vi "save data.vi"(8 "backwashing?":bool, 9 "coagulant dose":dbl) -> ()   [LabVIEW 2019]
uses:
  data buffer cmd.ctl
  file paths.ctl
panel:
  out "data labels":string[](array[string])
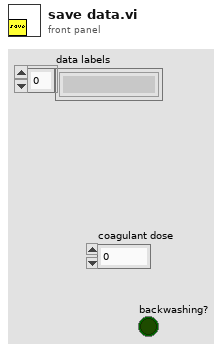
[diagram p1: front panel]
types:
  T1 = typedef "file paths.ctl" = enum16{"read paths", "close"}
  T2 = typedef "data buffer cmd.ctl" = enum16{"set buffer size", "write", "refill buffer", "read recent", "read all", "clear"}
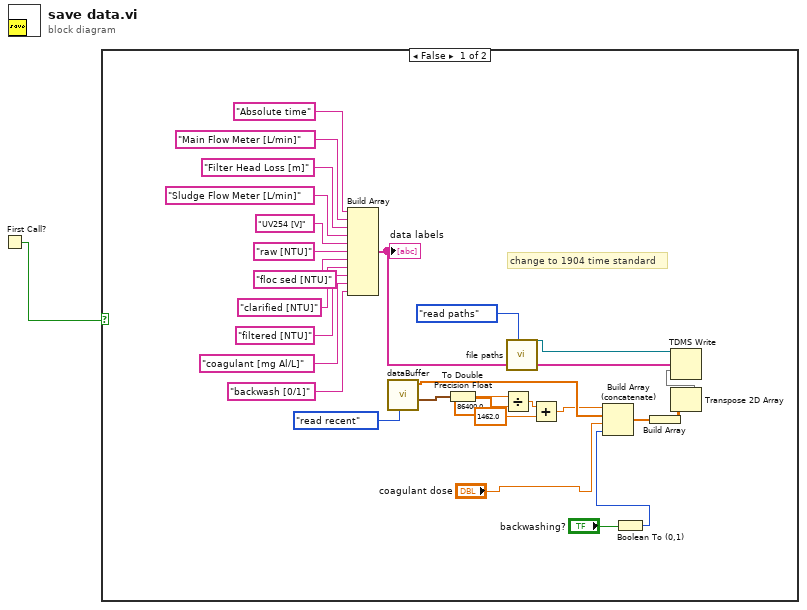
[diagram p0: block diagram]
diagram:
  n1 = First Call?() -> (First Call?: T/F=w1:bool)
  n2 = case shown="False" w1 {
    frame False {
      # "change to 1904 time standard"
      n3 = Build Array("Absolute time", "Main Flow Meter [L/min]", "Filter Head Loss [m]", "Sludge Flow Meter [L/min]", "UV254 [V]" ("element"), "raw [NTU]", "floc sed [NTU]", "clarified [NTU]", "filtered [NTU]" ("element"), "coagulant [mg Al/L]" ("element"), "backwash [0/1]" ("element")) -> (w17:string[])
      "data labels" <- w17
      n4 = call "dataBuffer.vi"("command"=data_buffer_cmd."read recent") -> ("recent time"=w13:timestamp, "recent data"=w16:dbl[])  [unwired: 5 in, 4 out]
      n5 = To Double Precision Float(number=w13) -> (double precision float=w8:dbl)
      n6 = Divide(x=w8, y=86400.0) -> (x/y=w6:dbl)
      n7 = call "file paths.vi"("file path control"=file_paths."read paths") -> ("datalog"=w29:refnum<k34>)  [unwired: 7 in, 3 out]
      n8 = Add(x=w6, y=1462.0) -> (x+y=w4:dbl)
      n9 = Boolean To (0,1)(Boolean="backwashing?") -> (0, 1=w14:i16)
      n10 = Build Array (concatenate)(w4, w16, "coagulant dose", w14) -> (w12:dbl[])
      n11 = Build Array(w12) -> (w10:dbl[][])
      n12 = Transpose 2D Array(2D array=w10) -> (transposed array=w9:dbl[][])
      n13 = TDMS Write(0:w29, 7:w17, 9:w9) -> ()  [unwired: 3 in, 4 out]
    }
    frame True {
    }
  }
